vi "Write to Text File.vi"(8 "error in":errorcluster, 10 "file path (use dialog)":path=path "C:/CoMP-S Observer/focus.txt", 11 "text":string) -> (0 "error out":errorcluster)   [LabVIEW 2014]
doc: "Writes simulated, timestamped data to a text file in ASCII format that can be read by spreadsheet applications.\nThe VI opens a new file or overwrites an existing file. It calls the subVI Acquire Data (Simulated).vi to generate a timestamped data array that contains (number of acquisition) sets of data, and its length is equal to (number of acquisitions)*(number of points/acquisition). The data is plotted on the graph one set at a time.\nThe VI also converts an array of data to a row of tab-separated columns, prepends to it the timestamp column, and terminates the row with the end of line character. Refer to the Read from Text File VI in this LLB and the spreadsheet examples for more file formats."
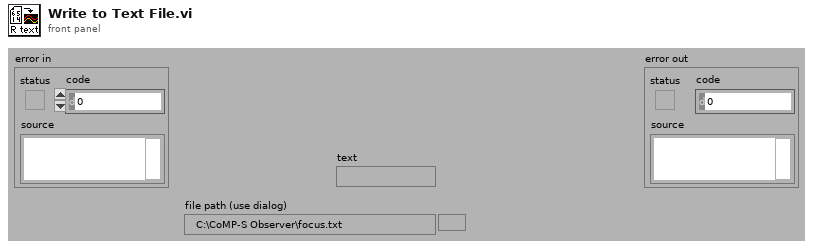
[diagram p1: front panel]
types:
  T1 = enum16{"open", "replace", "create", "open or create", "replace or create", "replace or create with confirmation"}
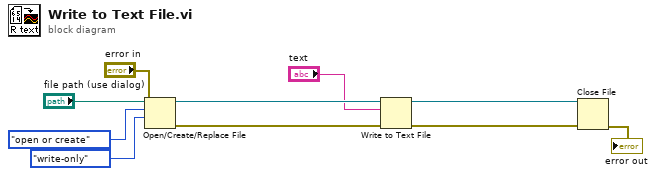
[diagram p0: block diagram]
diagram:
  n1 = Open/Create/Replace File(file path (use dialog)="file path (use dialog)", error in="error in", operation (0:open)=T1."open or create", access (0:read/write)=enum16{"read/write", "read-only", "write-only"}."write-only") -> (refnum out=w7:refnum<file>, error out=w6:errorcluster)  [unwired: 3 out]
  n2 = Write to Text File(file (use dialog)=w7, text="text", error in=w6) -> (refnum out=w10:refnum<file>, error out=w9:errorcluster)  [unwired: 1 in, 1 out]
  n3 = Close File(refnum=w10, error in=w9) -> (error out=→"error out":errorcluster)  [unwired: 1 out]
